vi "Start Lock-In Channel.vi"(7 "index":i32, 8 "error in":errorcluster, 10 "config":cluster{"config":T1, "record length":u32}, 11 "host in":refnum<class "LIA Host Interface FPGA.lvclass">) -> (0 "error out":errorcluster, 3 "host out":refnum<class "LIA Host Interface FPGA.lvclass">)   [LabVIEW 2017, in "LIA Host Interface FPGA.lvclass"]
uses:
  LIA Host Interface FPGA.lvclass
  host/Public/lock-in settings.ctl
  Properties/FpgaSession_GET.vi
  host/Lock-In Amplifier Example Host.lvlib
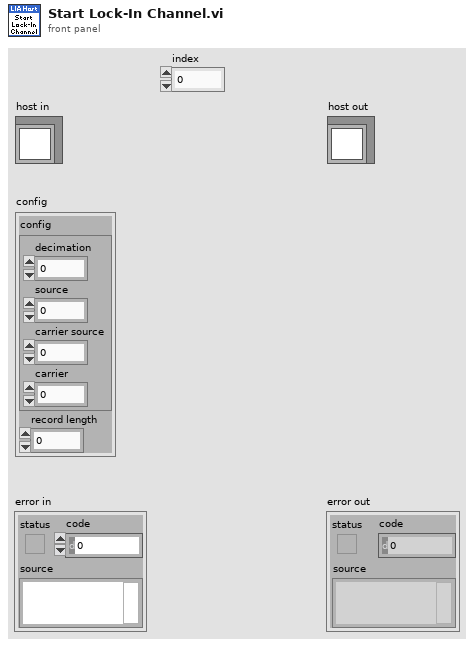
[diagram p1: front panel]
types:
  T1 = typedef "Lock-In Amplifier Example Host.lvlib/lock-in settings.ctl" = cluster{"decimation":i32, "source":i32, "carrier source":i32, "carrier":dbl}
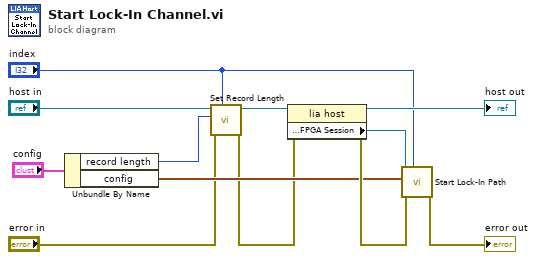
[diagram p0: block diagram]
diagram:
  n1 = Unbundle By Name("config") -> ("record length"=w1:u32, "config"=w7:T1)
  n2 = call "Set Record Length.vi"("instance"="index", "error in"="error in", "record length"=w1, "lia host in"="host in") -> ("error out"=w3:errorcluster, "lia host out"=w5:refnum<class "LIA Host Interface FPGA.lvclass">)  [unwired: 6 in]
  n3 = property class="lia host"(reference=w5, error in=w3) -> (reference out=→"host out":refnum<class "LIA Host Interface FPGA.lvclass">, error out=w9:errorcluster, "Properties:FPGA Session"=w11:refnum<k20>)
  n4 = call "Start Lock-In Path.vi"("instance"="index", "error in"=w9, "config"=w7, "fpga session in"=w11) -> ("error out"=→"error out":errorcluster)  [unwired: 6 in, 1 out]
